vi "Wiimote Battery.vi"(8 "error in (no error)":errorcluster, 9 "Wiimote Player #":i32=1, 11 "LV WiiMote Interface In":T1) -> (0 "error out":errorcluster, 1 "BatteryRaw":u8, 2 "Battery":sgl, 3 "LV WiiMote Interface out":T1)   [LabVIEW 2012, in "LV Wiimote Interface.lvclass"]
uses:
  LV Wiimote Interface.lvclass
  Controls/LV Wiimote Interface.ctl
  C:/Program Files/National Instruments/LabVIEW 2012/vi.lib/LabVIEW Hacker/WiiMote/Dependencies/WiimoteLib.dll
  Program Files/National Instruments/LabVIEW 2012/vi.lib/LabVIEW Hacker/WiiMote/Dependencies/WiimoteLib.dll
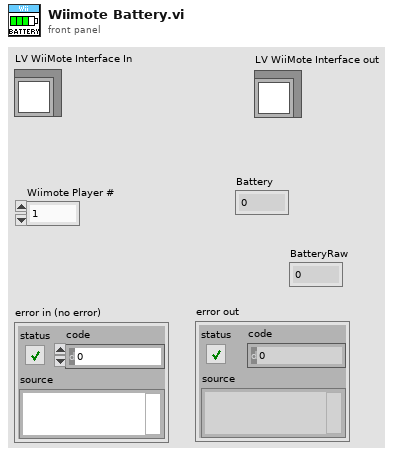
[diagram p1: front panel]
types:
  T1 = typedef "LV Wiimote Interface.ctl" = refnum<class "LV Wiimote Interface.lvclass">
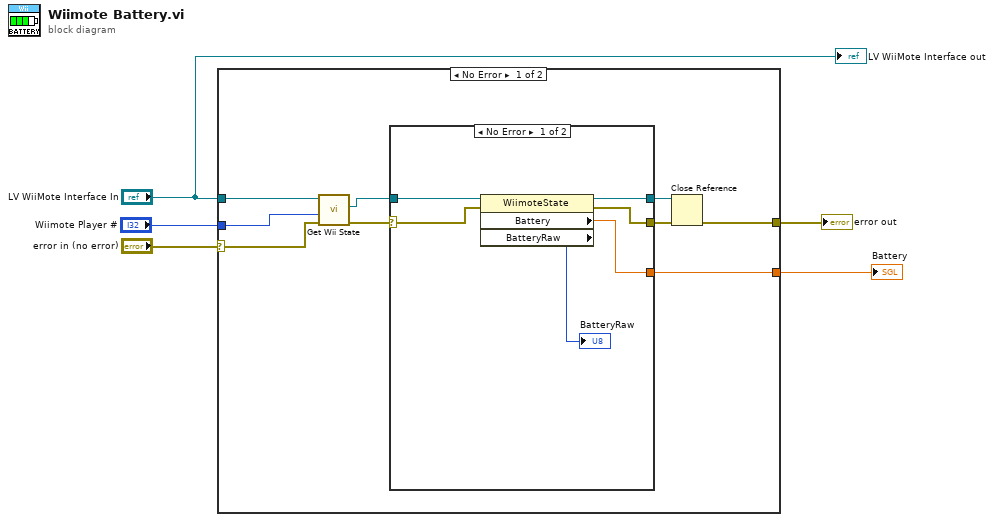
[diagram p0: block diagram]
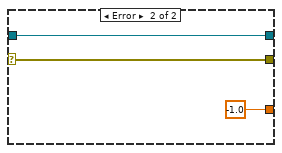
[diagram p2: hidden frame]
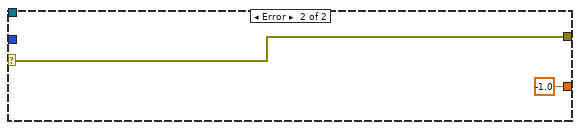
[diagram p3: hidden frame]
diagram:
  n1 = case shown="No Error" "error in (no error)" {
    selector: "error in (no error)" -> [w13 w25]
    tunnel: "LV WiiMote Interface In" -> [w14 _]
    tunnel: "Wiimote Player #" -> [w8 _]
    tunnel: [w10 w25] -> w2
    tunnel: [w7 sgl -1.0 ("Battery")] -> w1
    frame No Error {
      n2 = call "Get Wii State.vi"("error in (no error)"=w13, "Wiimote Player #"=w8, "LV Wiimote Interface in"=w14) -> ("error out"=w12:errorcluster, "WiimoteState"=w6:refnum<k24>)  [unwired: 6 in, 1 out]
      n3 = case shown="No Error" w12 {
        selector: w12 -> [w19 w23]
        tunnel: w6 -> [w20 w22]
        tunnel: [w16 w23] -> w11
        tunnel: [w18 w22] -> w9
        tunnel: [w17 sgl -1.0 ("Battery")] -> w7
        frame No Error {
          n4 = property class="WiimoteState"(reference=w20, error in=w19) -> (reference out=w18:refnum<k24>, error out=w16:errorcluster, "Battery"=w17:sgl, "BatteryRaw"=→"BatteryRaw":u8)
        }
        frame Error {
        }
      }
      n5 = Close Reference(reference=w9, error in (no error)=w11) -> (error out=w10:errorcluster)
    }
    frame Error {
    }
  }
  "error out" <- w2
  "Battery" <- w1
  "LV WiiMote Interface out" <- "LV WiiMote Interface In"
